vi "Main.vi"(8 "error in":errorcluster, 11 "ChartView in":refnum<class "ChartView.lvclass">) -> (0 "error out":errorcluster, 3 "ChartView out":refnum<class "ChartView.lvclass">)   [LabVIEW 2020, in "ChartView.lvclass"]
doc: "The <b>Queued Message Handler</b> of the Worker that owns this VI."
uses:
  ChartView.lvclass
  C:/Program Files (x86)/National Instruments/LabVIEW 2020/vi.lib/addons/_Workers/Library/Classes/Worker/Worker.lvclass
  ChartView.lvclass/ChartView.ctl
  Initialization Data.ctl
  Response Cases.ctl
  rqp_Update Chart Data.ctl
  <vilib>/addons/_Workers/Library/Classes/Message Queue/Message Queue.lvclass
  DAQ Worker/DAQ Worker.lvclass
panel:
  out "波形图表":dbl(graph)
  in  "START STOP":enum32{"Start", "Stop"}(radio)
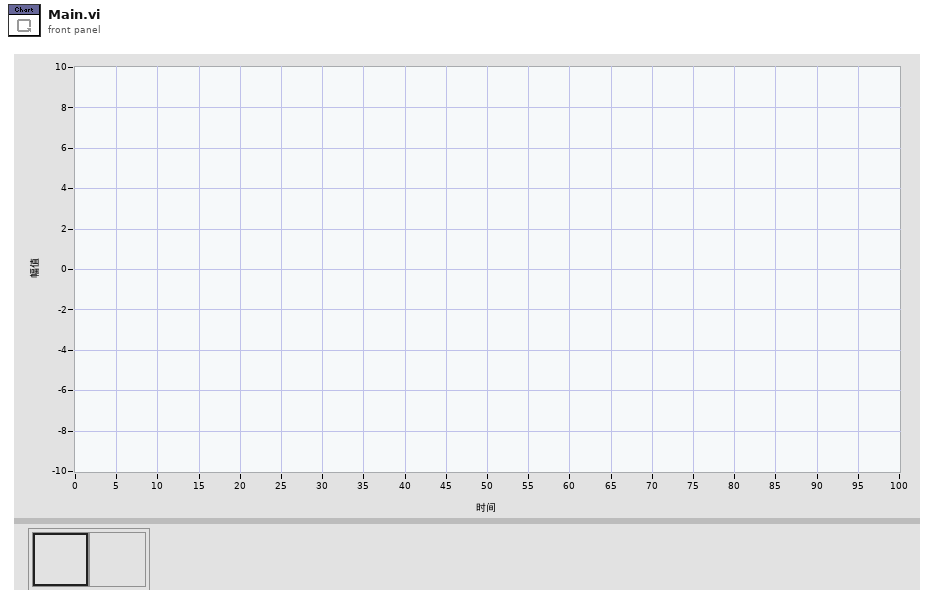
[diagram p1: front panel]
types:
  T1 = typedef "ChartView.lvclass/Initialization Data.ctl" = cluster{"Response Cases":T2}
  T2 = typedef "ChartView.lvclass/Response Cases.ctl" = cluster{"Placeholder - Can be deleted":string}
  T3 = typedef "ChartView.lvclass/rqp_Update Chart Data.ctl" = cluster{"Data":dbl}
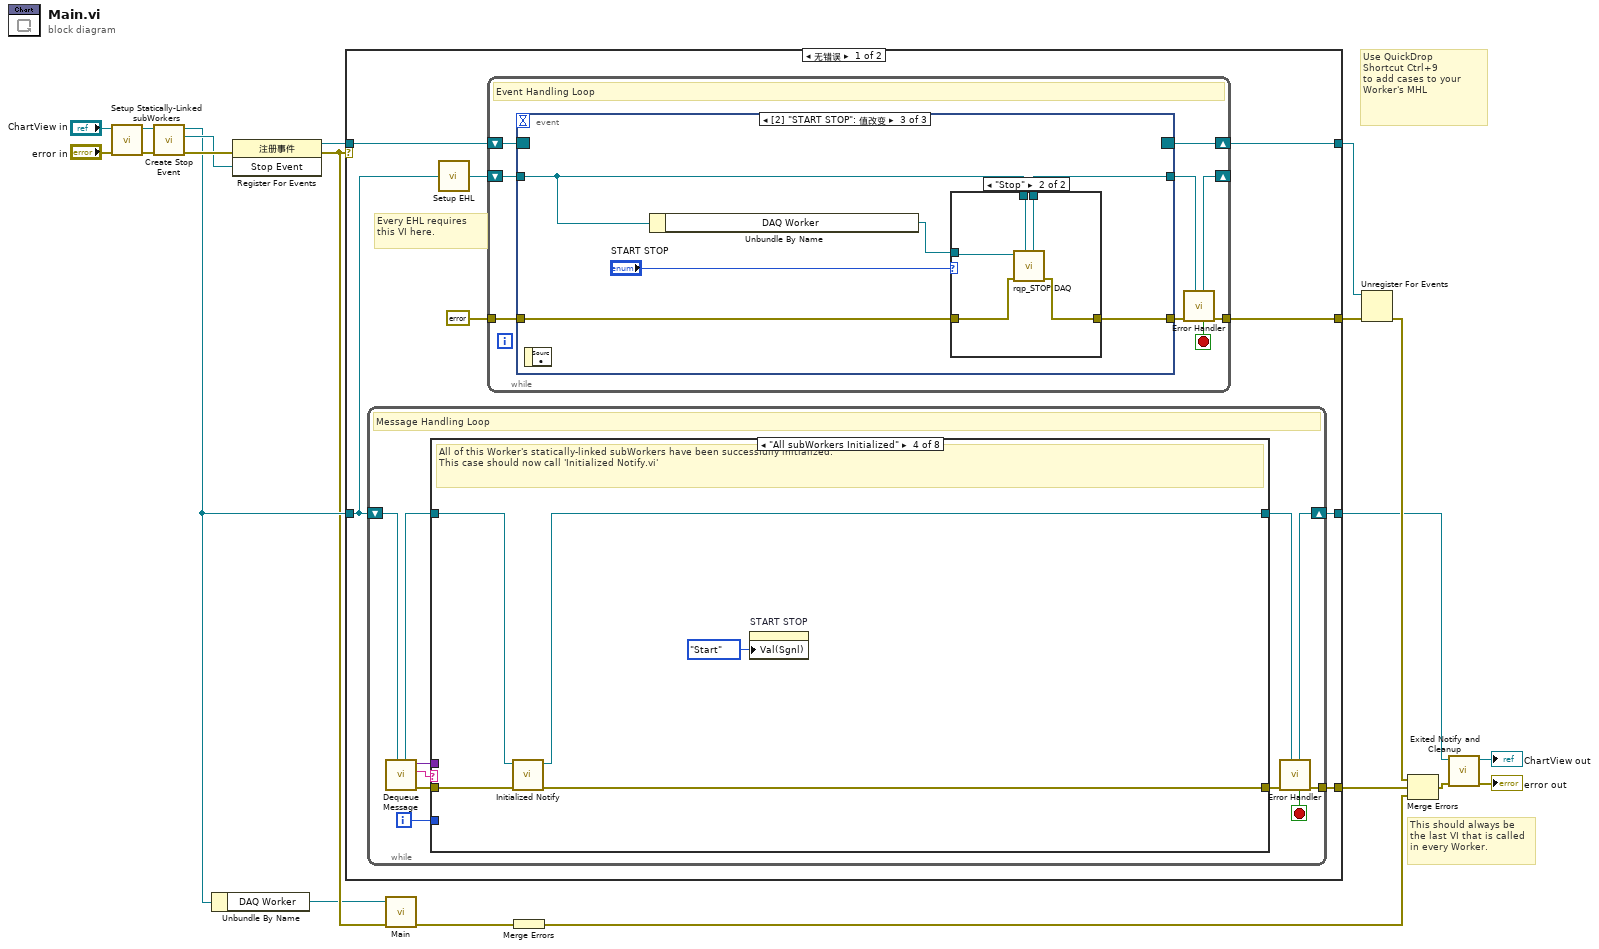
[diagram p0: block diagram]
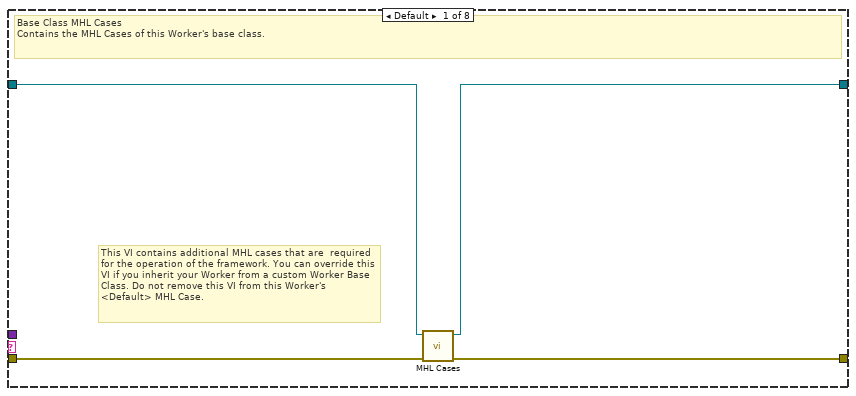
[diagram p2: hidden frame]
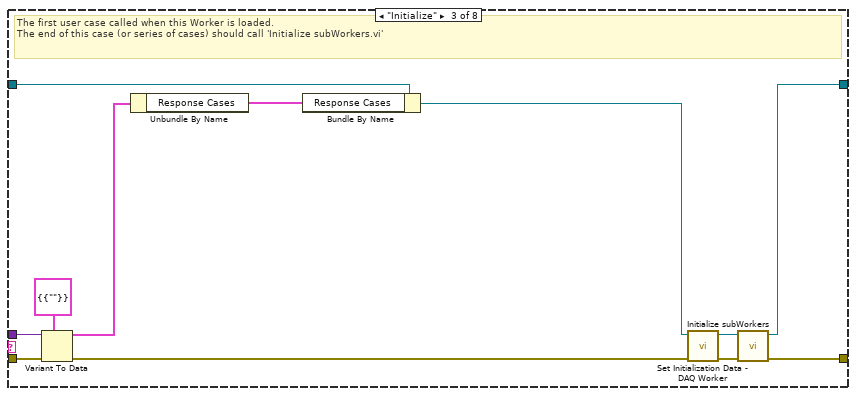
[diagram p4: hidden frame]
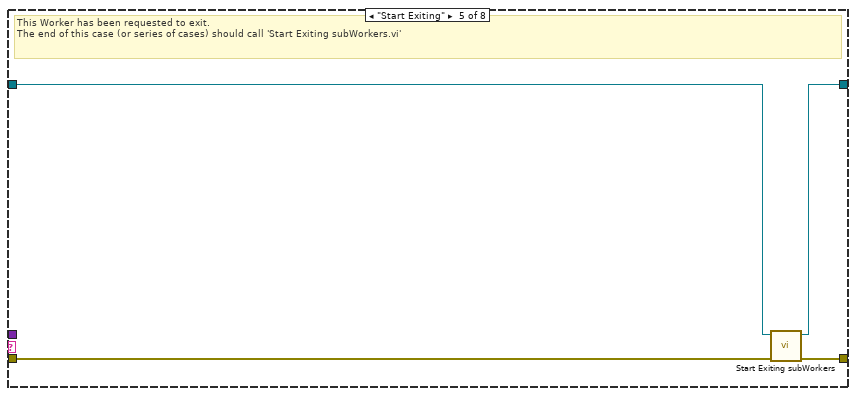
[diagram p5: hidden frame]
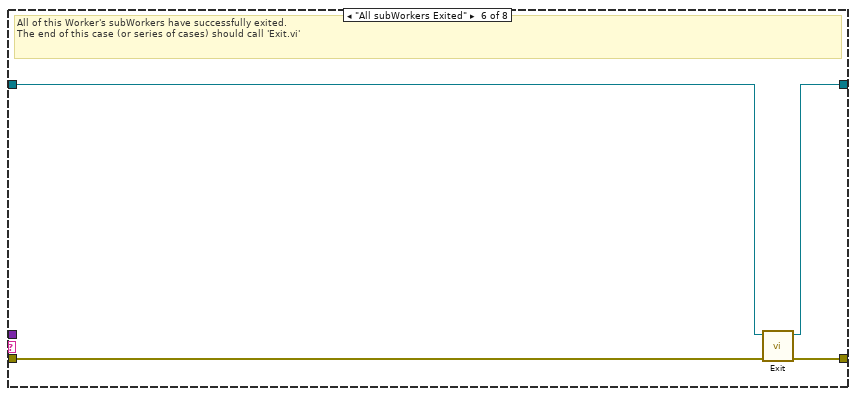
[diagram p6: hidden frame]
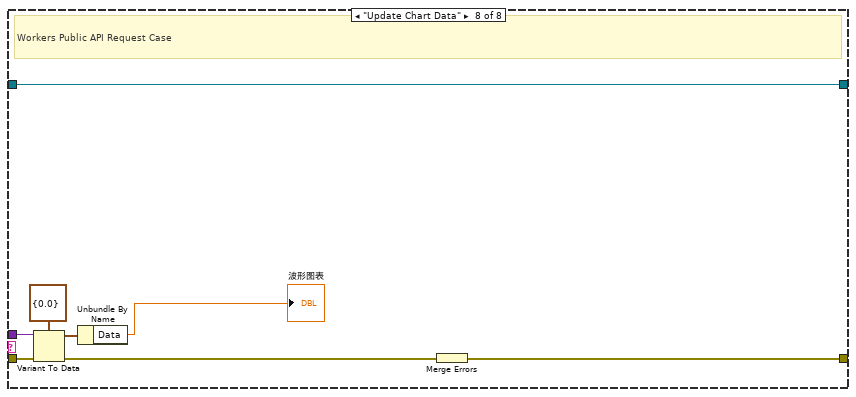
[diagram p8: hidden frame]
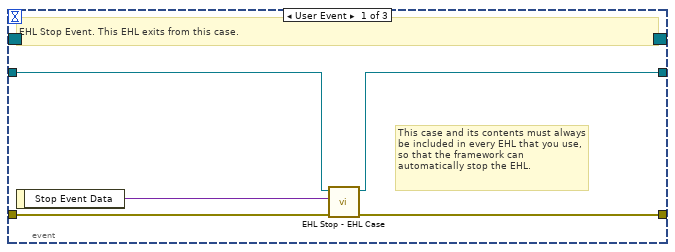
[diagram p9: hidden frame]
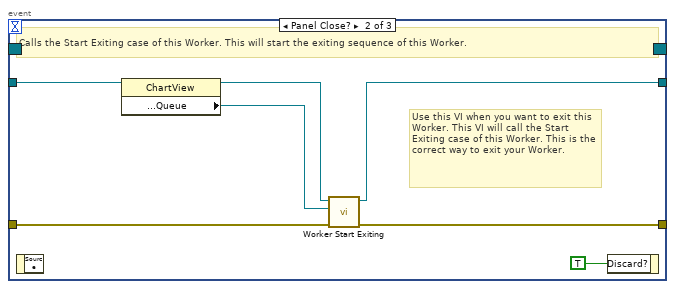
[diagram p10: hidden frame]
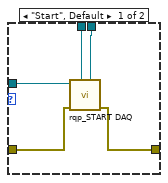
[diagram p11: hidden frame]
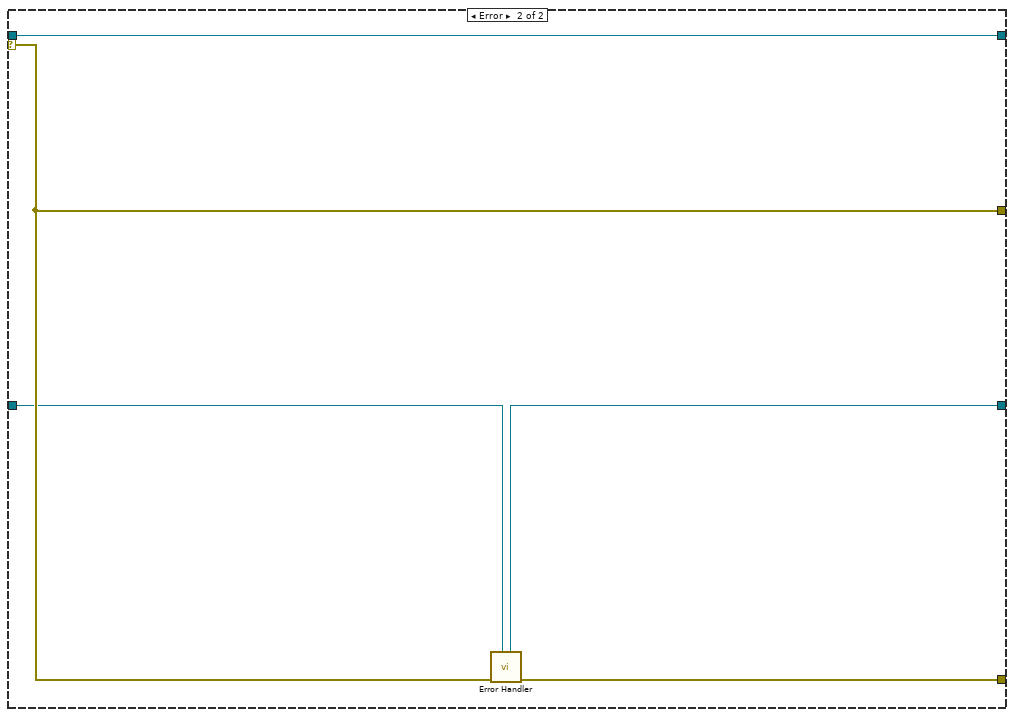
[diagram p12: hidden frame]
diagram:
  # "Use QuickDrop\nShortcut Ctrl+9\nto add cases to your\nWorker's MHL"
  # "This should always be the last VI that is called in every Worker."
  n1 = call "Setup Statically-Linked subWorkers.vi"("error in"="error in", "ChartView in"="ChartView in") -> ("error out"=w6:errorcluster, "ChartView out"=w4:refnum<class "ChartView.lvclass">)  [unwired: 8 in]
  n2 = call-dynamic "Create Stop Event.vi"("error in"=w6, "Worker"=w4) -> ("error out"=w15:errorcluster, "Stop Event"=w12:refnum<user-event>, "Worker out"=w9:refnum<class "ChartView.lvclass">)  [unwired: 7 in]
  n3 = Unbundle By Name(w9) -> ("DAQ Worker"=w1:refnum<class "DAQ Worker.lvclass">)
  n4 = register-events(error in=w15, w12) -> (reference out=w14:refnum<event-registration>, error out=w7:errorcluster)  [unwired: 1 in]
  n5 = case shown="无错误" w7 {
    tunnel: w9 -> [w23 w119]
    tunnel: [w21 w120] -> w13
    tunnel: w14 -> [w28 w121]
    tunnel: [w25 w122] -> w19
    tunnel: [w27 w121] -> w18
    tunnel: [w22 w118] -> w16
    selector: w7 -> [_ w122]
    frame No Error {
      # "Every EHL requires\nthis VI here."
      n6 = while {
        shift-right: [w37] -> w22
        shift-left: w23 -> [w39]
        tunnel: [w38] -> w21
        i -> [w30]
        stop <- w31 stop-if-true
        # "Message Handling Loop"
        n7 = call-dynamic "Dequeue Message.vi"("Worker"=w39) -> ("error out"=w36:errorcluster, "Case out"=w32:string, "Data out"=w29:variant, "Worker out"=w34:refnum<class "ChartView.lvclass">)  [unwired: 6 in, 1 out]
        n8 = case "Worker MHL Case Structure (DO NOT CHANGE LABEL NAME)" shown="\"All subWorkers Initialized\"" w32 {
          tunnel: w36 -> [w43 w44 w55 w60 w63 w70 w72 w79]
          tunnel: [w42 w44 w57 w59 w66 w69 w72 w74] -> w35
          tunnel: w34 -> [w41 w45 w54 w62 w64 w68 w71 w80]
          tunnel: [w40 w45 w56 w61 w65 w67 w71 w80] -> w33
          tunnel: w30 -> [_ _ _ _ _ _ _ _]
          tunnel: w29 -> [_ _ w52 _ _ _ _ w76]
          frame Default {
            # "This VI contains additional MHL cases that are  required for the operation of the framework. You can override this VI if you inherit your Worker from a custom Worker Base Class. Do not remove this VI from this Worker's <Default> MHL Case."
            # "Base Class MHL Cases\nContains the MHL Cases of this Worker's base class."
            n9 = call-dynamic "MHL Cases.vi"("error in"=w43, "BaseView in"=w41) -> ("error out"=w42:errorcluster, "BaseView out"=w40:refnum<class "ChartView.lvclass">)  [unwired: 8 in]
          }
          frame "------------ FRAMEWORK CASES -----------" {
            # "Start of Workers Framework Cases"
          }
          frame "Initialize" {
            # "The first user case called when this Worker is loaded.\nThe end of this case (or series of cases) should call 'Initialize subWorkers.vi'"
            n10 = Variant To Data(error in=w55, type=T1 {"Response Cases"={"Placeholder - Can be deleted"=""}} ("Initialization Data"), Variant=w52) -> (data=w51:T1, error out=w53:errorcluster)
            n11 = Unbundle By Name(w51) -> ("Response Cases"=w50:T2)
            n12 = Bundle By Name ("按名称捆绑")(cluster=w54, "Response Cases"=w50) -> (w46:refnum<class "ChartView.lvclass">)
            n13 = call "Set Initialization Data - DAQ Worker.vi"("error in"=w53, "ChartView in"=w46) -> ("error out"=w48:errorcluster, "ChartView out"=w47:refnum<class "ChartView.lvclass">)  [unwired: 8 in]
            n14 = call-dynamic "Initialize subWorkers.vi"("error in"=w48, "Worker"=w47) -> ("error out"=w57:errorcluster, "dup Worker out"=w56:refnum<class "ChartView.lvclass">)  [unwired: 8 in]
          }
          frame "All subWorkers Initialized" {
            # "All of this Worker's statically-linked subWorkers have been successfully initialized.\nThis case should now call 'Initialized Notify.vi'"
            n15 = call-dynamic "Initialized Notify.vi"("error in"=w60, "Worker"=w62) -> ("error out"=w59:errorcluster, "dup Worker out"=w61:refnum<class "ChartView.lvclass">)  [unwired: 8 in]
            n16 = property on="START STOP" class="RadioBtnsControl (严格)"("Val(Sgnl)"=enum32{"Start", "Stop"}."Start" ("值(信号)")) -> ()  [unwired: 2 in, 2 out]
          }
          frame "Start Exiting" {
            # "This Worker has been requested to exit. \nThe end of this case (or series of cases) should call 'Start Exiting subWorkers.vi'"
            n17 = call-dynamic "Start Exiting subWorkers.vi"("error_in"=w63, "Worker"=w64) -> ("error out"=w66:errorcluster, "dup Worker out"=w65:refnum<class "ChartView.lvclass">)  [unwired: 8 in]
          }
          frame "All subWorkers Exited" {
            # "All of this Worker's subWorkers have successfully exited. \nThe end of this case (or series of cases) should call 'Exit.vi'"
            n18 = call-dynamic "Exit.vi"("error_in"=w70, "Worker"=w68) -> ("error out"=w69:errorcluster, "dup Worker out"=w67:refnum<class "ChartView.lvclass">)  [unwired: 8 in]
          }
          frame "------------- PUBLIC API CASES -------------" {
            # "Start of Workers Public API Cases"
          }
          frame "Update Chart Data" {
            # "Workers Public API Request Case"
            n19 = Variant To Data(error in=w79, type=T3 {"Data"=0.0} ("Data"), Variant=w76) -> (data=w75:T3, error out=w78:errorcluster)
            n20 = Unbundle By Name(w75) -> ("Data"=→"波形图表":dbl)
            n21 = Merge Errors(w78) -> (w74:errorcluster)
          }
        }
        n22 = call-dynamic "Error Handler.vi"("Worker"=w33, "error_in"=w35) -> ("error out"=w38:errorcluster, "Stop Loop"=w31:bool, "Worker out"=w37:refnum<class "ChartView.lvclass">)  [unwired: 7 in]
      }
      n23 = call-dynamic "Setup EHL.vi"("Worker"=w23) -> ("Worker out"=w24:refnum<class "ChartView.lvclass">)  [unwired: 14 in]
      n24 = while "Event Handling Loop" {
        shift-right: [w89] -> w27
        shift-left: w28 -> [w88]
        tunnel: [w84] -> w25
        tunnel: errorcluster {"status"=FALSE, "code"=0, "source"=""} ("error constant") -> [w86]
        shift-right: [w82] -> _
        shift-left: w24 -> [w87]
        stop <- w81 stop-if-true
        # "Event Handling Loop"
        n25 = event shown="[2] \"START STOP\": 值改变" {
          selector: w88 -> [_ _ _]
          dyn-events: [_ _ _] -> w89
          timeout: _ -> [_ _ _]
          tunnel: [w93 w100 w104] -> w85
          tunnel: w86 -> [w94 w99 w105]
          tunnel: w87 -> [w92 w98 w103]
          tunnel: [w91 w97 w102] -> w83
          event User Event {
            # "This case and its contents must always be included in every EHL that you use, so that the framework can automatically stop the EHL."
            # "EHL Stop Event. This EHL exits from this case."
            n26 = event-data() -> ("Stop Event Data"=w90:variant)  [unwired: 1 in]
            n27 = call-dynamic "EHL Stop - EHL Case.vi"("error in"=w94, "Stop Event Data"=w90, "Worker"=w92) -> ("error out"=w93:errorcluster, "Worker out"=w91:refnum<class "ChartView.lvclass">)  [unwired: 7 in]
          }
          event Panel Close? {
            # "Use this VI when you want to exit this Worker. This VI will call the Start Exiting case of this Worker. This is the correct way to exit your Worker."
            # "Calls the Start Exiting case of this Worker. This will start the exiting sequence of this Worker."
            n28 = event-data() -> ()  [unwired: 1 in, 1 out]
            n29 = property class="ChartView"(reference=w98) -> (reference out=w96:refnum<class "ChartView.lvclass">, "Accessors:Read:Public API:Queue"=w95:refnum<class "Message Queue.lvclass">)  [unwired: 1 in, 1 out]
            n30 = call-dynamic "Worker Start Exiting.vi"("error_in"=w99, "Message Queue"=w95, "Worker"=w96) -> ("error out"=w100:errorcluster, "dup Worker out"=w97:refnum<class "ChartView.lvclass">)  [unwired: 7 in]
            n31 = event-data ("事件过滤节点")("Discard?"=TRUE) -> ()  [unwired: 1 in, 1 out]
          }
          event "START STOP": Value Change {
            n32 = event-data() -> ()  [unwired: 1 in, 1 out]
            n33 = Unbundle By Name(w103) -> ("DAQ Worker"=w106:refnum<class "DAQ Worker.lvclass">)
            n34 = case shown="\"Stop\"" "START STOP" {
              tunnel: w106 -> [w112 w115]
              tunnel: w105 -> [w111 w113]
              tunnel: [w110 w114] -> w104
              tunnel: w103 -> [w109 w117]
              tunnel: [w108 w116] -> w102
              frame "Start", Default {
                n35 = call "rqp_START DAQ.vi"("Caller in"=w109, "error in"=w111, "DAQ Worker in"=w112) -> ("error out"=w110:errorcluster, "dup Caller out"=w108:refnum<class "ChartView.lvclass">)  [unwired: 6 in, 1 out]
              }
              frame "Stop" {
                n36 = call "rqp_STOP DAQ.vi"("Caller in"=w117, "error in"=w113, "DAQ Worker in"=w115) -> ("error out"=w114:errorcluster, "dup Caller out"=w116:refnum<class "ChartView.lvclass">)  [unwired: 6 in, 1 out]
              }
            }
          }
        }
        n37 = call-dynamic "Error Handler.vi"("Worker"=w83, "error_in"=w85) -> ("error out"=w84:errorcluster, "Stop Loop"=w81:bool, "Worker out"=w82:refnum<class "ChartView.lvclass">)  [unwired: 7 in]
      }
    }
    frame Error {
      n38 = call-dynamic "Error Handler.vi"("Worker"=w119, "error_in"=w122) -> ("error out"=w120:errorcluster, "Worker out"=w118:refnum<class "ChartView.lvclass">)  [unwired: 7 in, 1 out]
    }
  }
  n39 = call-dynamic "Main.vi"("error in"=w7, "DAQ Worker in"=w1) -> ("error out"=w3:errorcluster)  [unwired: 8 in, 1 out]
  n40 = Merge Errors(w3) -> (w2:errorcluster)
  n41 = Unregister For Events(event registration refnum=w18, error in=w19) -> (error out=w20:errorcluster)
  n42 = Merge Errors ("合并错误")(w20, w13, w2) -> (w17:errorcluster)
  n43 = call-dynamic "Exited Notify and Cleanup.vi"("error_in"=w17, "Worker"=w16) -> ("error out"=→"error out":errorcluster, "dup Worker out"=→"ChartView out":refnum<class "ChartView.lvclass">)  [unwired: 8 in]
